vi "Run GraphViz.vi"(11 "output to graphviz":string) -> (2 "new picture":picture, 3 "Unique Temporary File Path":path)   [LabVIEW 2015, in "GraphViz Mapping Visualizer.lvlib"]
doc: "Create Temporary Files and Call GraphViz to create image and load into picture control."
uses:
  GraphViz Mapping Visualizer.lvlib
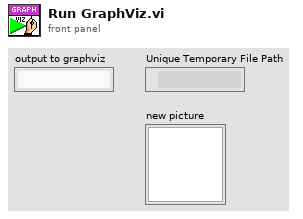
[diagram p1: front panel]
types:
  T1 = enum16{"open", "replace", "create", "open or create", "replace or create", "replace or create with confirmation"}
  T2 = typedef "imagedata.ctl" = cluster{"image type":i32, "image depth":i32, "image":u8[], "mask":u8[], "colors":u32[], "Rectangle":cluster{"left":i16, "top":i16, "right":i16, "bottom":i16}}
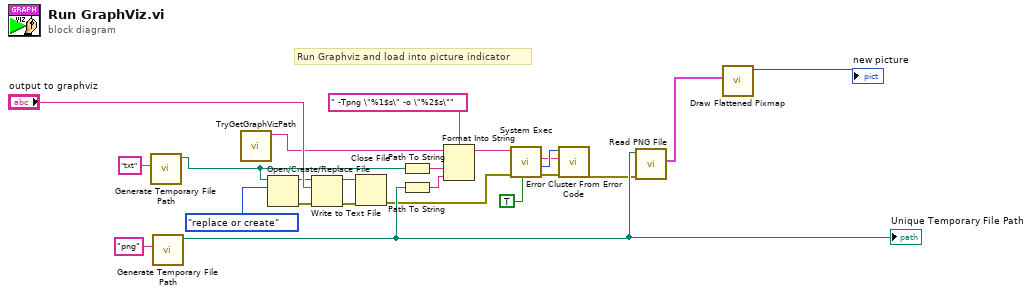
[diagram p0: block diagram]
diagram:
  # "Run Graphviz and load into picture indicator"
  n1 = call <vilib>:"Generate Temporary File Path.vi"("Temporary File Extension (tmp)"="txt") -> ("Unique Temporary File Path"=w17:path)  [unwired: 9 in, 1 out]
  n2 = call <vilib>:"Generate Temporary File Path.vi"("Temporary File Extension (tmp)"="png") -> ("Unique Temporary File Path"=w20:path)  [unwired: 9 in, 1 out]
  "Unique Temporary File Path" <- w20
  n3 = call <vilib>:"TryGetGraphVizPath.vi"() -> ("Path"=w15:string)  [unwired: 10 in, 1 out]
  n4 = Open/Create/Replace File(file path (use dialog)=w17, operation (0:open)=T1."replace or create") -> (refnum out=w2:refnum<file>, error out=w3:errorcluster)  [unwired: 4 in, 1 out]
  n5 = Write to Text File(file (use dialog)=w2, text="output to graphviz", error in=w3) -> (refnum out=w5:refnum<file>, error out=w4:errorcluster)  [unwired: 1 in, 1 out]
  n6 = Close File(refnum=w5, error in=w4) -> (error out=w6:errorcluster)  [unwired: 1 out]
  n7 = Path To String(path=w17) -> (string=w12:string)
  n8 = Path To String(path=w20) -> (string=w14:string)
  n9 = Format Into String(format string=" -Tpng \"%1$s\" -o \"%2$s\"" ("name or relative path"), initial string=w15, w12, w14) -> (resulting string=w13:string)  [unwired: 1 in, 1 out]
  n10 = call <vilib>:"System Exec.vi"("run minimized? (F)"=TRUE, "error in (no error)"=w6, "command line"=w13) -> ("error out"=w8:errorcluster, "return code"=w10:i32, "standard error"=w9:string)  [unwired: 5 in, 1 out]
  n11 = call <vilib>:"Error Cluster From Error Code.vi"("error in (no error)"=w8, "error message (\"\")"=w9, "error code (0)"=w10) -> ("error out"=w19:errorcluster)  [unwired: 6 in]
  n12 = call <vilib>:"Read PNG File.vi"("error in (no error)"=w19, "path to PNG file"=w20) -> ("image data"=w22:T2)  [unwired: 7 in, 2 out]
  n13 = call <vilib>:"Draw Flattened Pixmap.vi"("image data"=w22) -> ("new picture"=→"new picture":picture)  [unwired: 8 in]
